vi "testGetErrorInfo.vi"(8 "error in (no error)":errorcluster) -> (0 "error out":errorcluster)   [LabVIEW 2018]
uses:
  <vilib>/addons/_JKI Toolkits/Caraya/classes/Assert/Assert Not Equal Value_Variant.vi
  <vilib>/addons/_JKI Toolkits/Caraya/classes/Test/Test.lvclass
  src/Logger/Logger.lvclass
  <vilib>/addons/_JKI Toolkits/Caraya/classes/Assert/Assert.lvclass
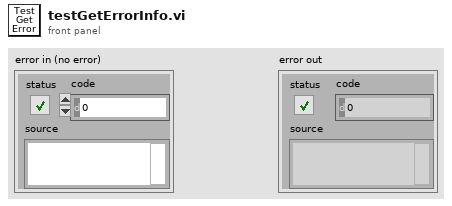
[diagram p1: front panel]
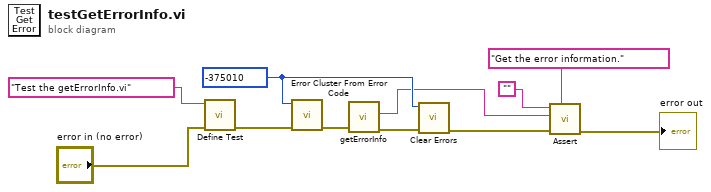
[diagram p0: block diagram]
diagram:
  w3 = -375010 ("error code (0)")
  n1 = call <vilib>:"Define Test.vi"("error in (no error)"="error in (no error)", "Label (VI Title)"="Test the getErrorInfo.vi") -> ("error out"=w9:errorcluster)  [unwired: 9 in]
  n2 = call <vilib>:"Error Cluster From Error Code.vi"("error in (no error)"=w9, "error code (0)"=w3) -> ("error out"=w8:errorcluster)  [unwired: 7 in]
  n3 = call "getErrorInfo.vi"("error in (no error)"=w8) -> ("error out"=w4:errorcluster, "infoErr"=w1:string)  [unwired: 8 in, 1 out]
  n4 = call <vilib>:"Clear Errors.vi"("error in (no error)"=w4, "specific error code to clear (0: all)"=w3) -> ("error out"=w2:errorcluster)  [unwired: 4 in, 1 out]
  n5 = call-poly <vilib>:"Assert.vi"("Label"="Get the error information.", "error in (no error)"=w2, "Y"=w1, "X"="") -> ("error out"=→"error out":errorcluster)  [unwired: 7 in]
